vi "2.vi"() -> ()   [LabVIEW 2014]
panel:
  out "error out 2":errorcluster
  out "error out":errorcluster
  in  "address":string
  out "TF":bool
  out "Boolean 2":bool
  in  "Call / Cancel":bool caption="Boolean"
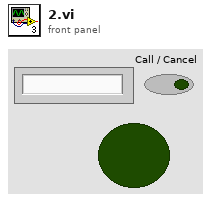
[diagram p1: front panel]
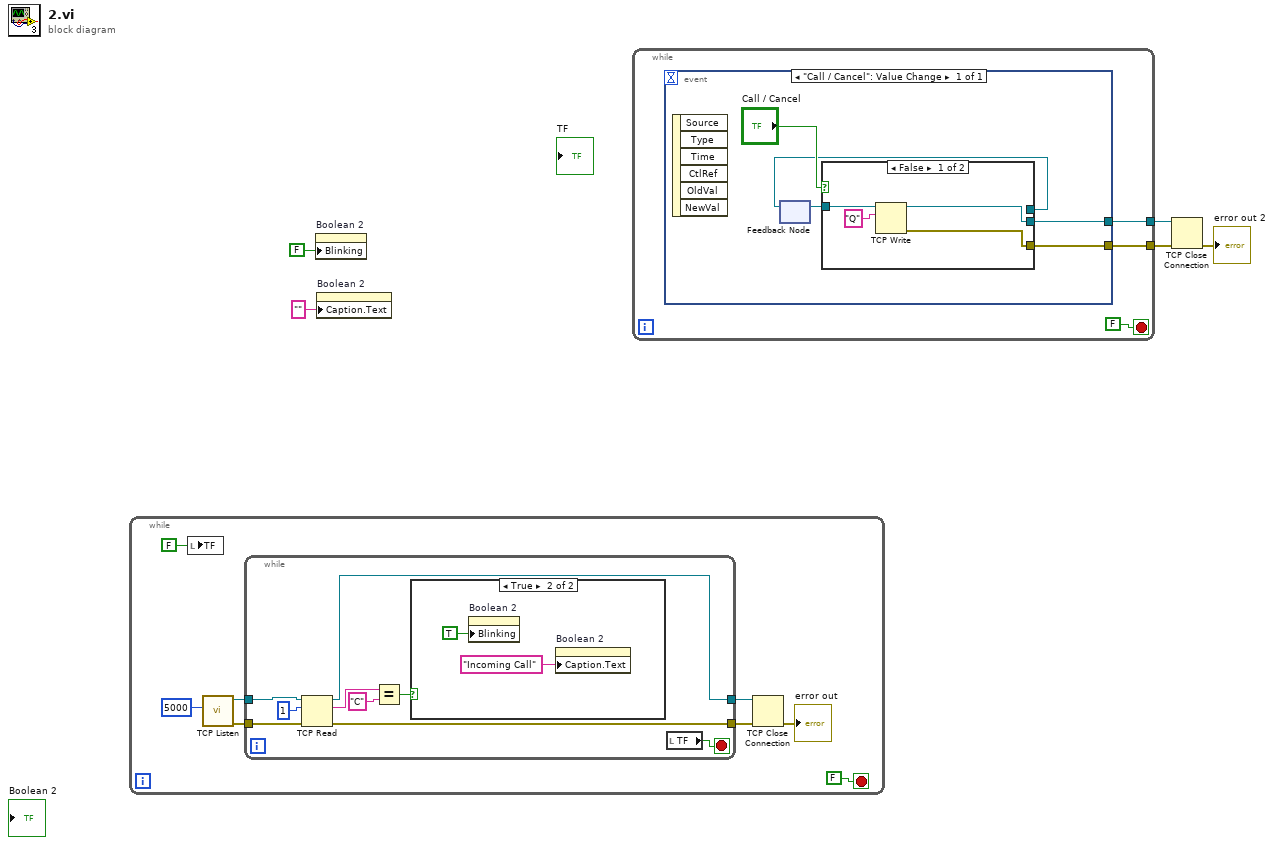
[diagram p0: block diagram]
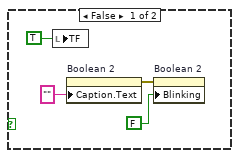
[diagram p2: hidden frame]
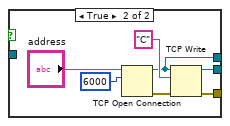
[diagram p3: hidden frame]
diagram:
  n1 = while {
    stop <- FALSE stop-if-true
    n2 = local write "TF"(FALSE ("TF")) -> ()
    n3 = call <vilib>:"TCP Listen.vi"("port"=u16 5000) -> ("error out"=w11:errorcluster, "connection ID"=w12:refnum<k5>)  [unwired: 6 in, 3 out]
    n4 = while {
      tunnel: w12 -> [w18]
      tunnel: w11 -> [w17]
      tunnel: [w14] -> w10
      tunnel: [w16] -> w9
      stop <- w15 stop-if-true
      n5 = TCP Read(connection ID=w18, bytes to read=1, error in (no error)=w17) -> (connection ID out=w14:refnum<k5>, data out=w21:string, error out=w16:errorcluster)  [unwired: 2 in]
      n6 = Equal?(x=w21, y="C") -> (x = y?=w20:bool)
      n7 = case shown="True" w20 {
        frame False {
          n8 = local write "TF"(TRUE ("TF")) -> ()
          n9 = property on="Boolean 2" class="Bool (strict)"("Caption.Text"="") -> (error out=w25:errorcluster)  [unwired: 2 in, 1 out]
          n10 = property on="Boolean 2" class="Bool (strict)"(error in=w25, "Blinking"=FALSE) -> ()  [unwired: 1 in, 2 out]
        }
        frame True {
          n11 = property on="Boolean 2" class="Bool (strict)"("Blinking"=TRUE) -> ()  [unwired: 2 in, 2 out]
          n12 = property on="Boolean 2" class="Bool (strict)"("Caption.Text"="Incoming Call") -> ()  [unwired: 2 in, 2 out]
        }
      }
      n13 = local read "TF"() -> (w15:bool)
    }
    n14 = TCP Close Connection(connection ID=w10, error in (no error)=w9) -> (error out=→"error out":errorcluster)  [unwired: 1 in, 1 out]
  }
  n15 = property on="Boolean 2" class="Bool (strict)"("Blinking"=FALSE) -> ()  [unwired: 2 in, 2 out]
  n16 = property on="Boolean 2" class="Bool (strict)"("Caption.Text"="") -> ()  [unwired: 2 in, 2 out]
  n17 = while {
    tunnel: [w30] -> w3
    tunnel: [w29] -> w2
    stop <- FALSE stop-if-true
    n18 = event shown="[0] \"Call / Cancel\": Value Change" {
      selector: _ -> [_]
      dyn-events: _ -> [_]
      timeout: _ -> [_]
      tunnel: [w36] -> w30
      tunnel: [w35] -> w29
      event "Call / Cancel": Value Change {
        n19 = event-data() -> ()  [unwired: 1 in, 6 out]
        n20 = feedback #1() -> (w32:refnum<k5>)  [unwired: 1 in]
        n21 = case shown="False" "Call / Cancel" {
          tunnel: [w39 w44] -> w36
          tunnel: [w38 w42] -> w35
          tunnel: [_ w41] -> w33
          tunnel: w32 -> [w37 _]
          frame False {
            n22 = TCP Write(connection ID=w37, data in="Q") -> (connection ID out=w39:refnum<k5>, error out=w38:errorcluster)  [unwired: 2 in, 1 out]
          }
          frame True {
            n23 = TCP Open Connection(address="address", remote port or service name=u16 6000) -> (connection ID=w41:refnum<k5>, error out=w45:errorcluster)  [unwired: 3 in]
            n24 = TCP Write(connection ID=w41, data in="C", error in (no error)=w45) -> (connection ID out=w44:refnum<k5>, error out=w42:errorcluster)  [unwired: 1 in, 1 out]
          }
        }
        n25 = feedback-in #1(w33) -> ()
      }
    }
  }
  n26 = TCP Close Connection(connection ID=w3, error in (no error)=w2) -> (error out=→"error out 2":errorcluster)  [unwired: 1 in, 1 out]
